vi "Plot Pole-Zero - cascade.vi"(4 "IIR Filter Cluster":T1) -> (1 "Pole-Zero Plot":cluster{dbl[], dbl[]}[](graph))   [LabVIEW 2016]
doc: "Plot the pole-zero diagram of a filter described by its cascade-form IIR filter cluster."
uses:
  <vilib>/Analysis/1siggen.llb/Ramp Pattern by Samples.vi
  <vilib>/Analysis/polynomials.llb/Remove Zero Coefficients (DBL).vi
  <vilib>/Analysis/polynomials.llb/Polynomial Roots (DBL).vi
  <vilib>/Analysis/NI_AALPro.lvlib
  <vilib>/Analysis/NI_AALBase.lvlib
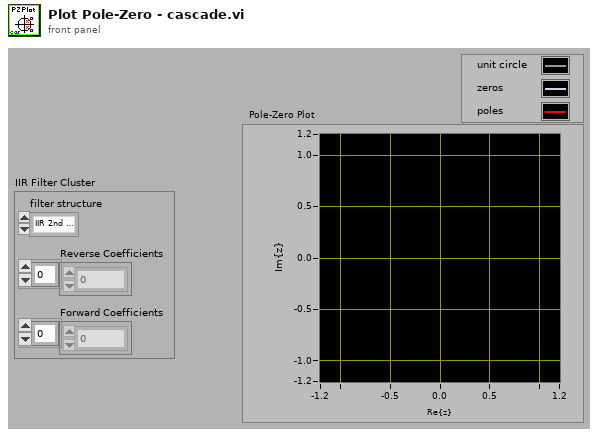
[diagram p1: front panel]
types:
  T1 = cluster{"filter structure":enum32{"IIR 2nd Order", "IIR 4th Order"}, "Reverse Coefficients":dbl[], "Forward Coefficients":dbl[]}
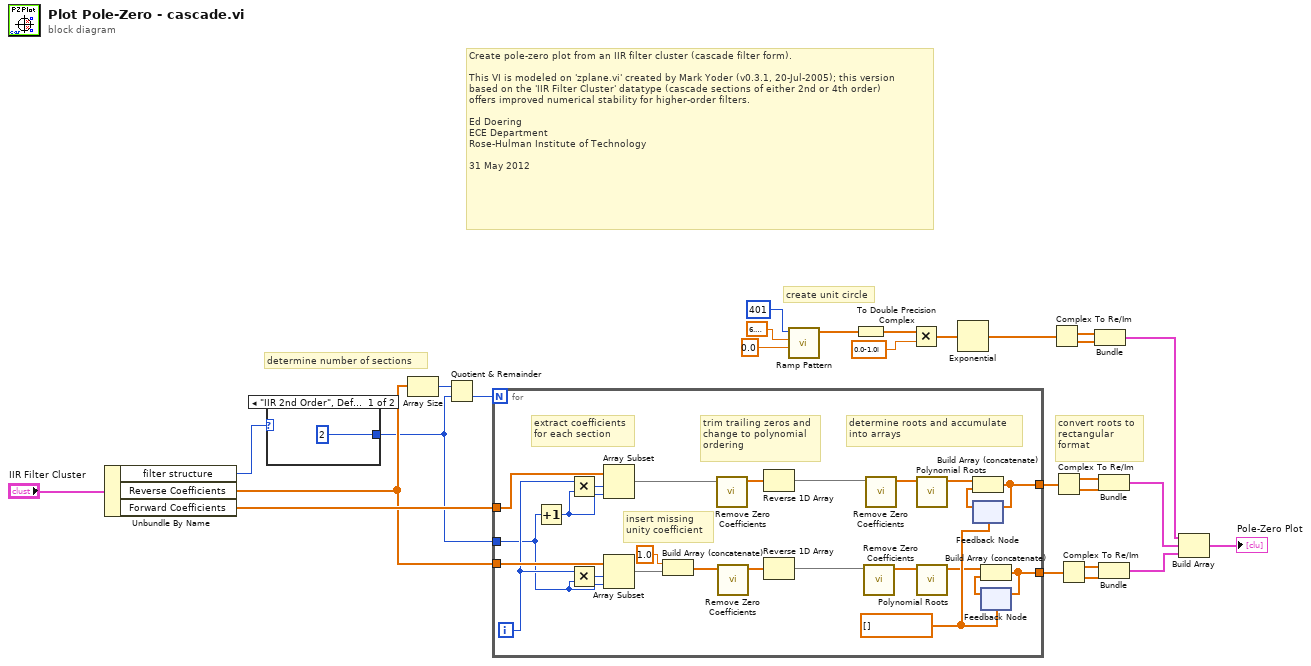
[diagram p0: block diagram]
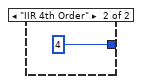
[diagram p2: hidden frame]
diagram:
  # "create unit circle"
  # "Create pole-zero plot from an IIR filter cluster (cascade filter form).\n\nThis VI is modeled on 'zplane.vi' created by Mark Yoder (v0.3.1, 20-Jul-2005); this version\nbased on the 'IIR Filter Cluster' datatype (cascade sections of either 2nd or 4th order)\noffers improved numerical stability for higher-order filters.\n\nEd Doering\nECE Department\nRose-Hulman Institute of Technology\n\n31 May 2012"
  # "convert roots to\nrectangular \nformat"
  # "determine number of sections"
  n1 = Unbundle By Name("IIR Filter Cluster") -> ("filter structure"=w19:enum32{"IIR 2nd Order", "IIR 4th Order"}, "Reverse Coefficients"=w21:dbl[], "Forward Coefficients"=w22:dbl[])
  n2 = case shown="\"IIR 2nd Order\", Default" w19 {
    tunnel: [2 ("y") 4 ("y")] -> w12
    frame "IIR 2nd Order", Default {
    }
    frame "IIR 4th Order" {
    }
  }
  n3 = Array Size(array=w21) -> (size(s)=w23:i32)
  n4 = Quotient & Remainder(x=w23, y=w12) -> (floor(x/y)=w20:i32)  [unwired: 1 out]
  n5 = for {
    N: w20 -> [_]
    tunnel: w22 -> [w52]
    tunnel: w21 -> [w50]
    tunnel: [w44] -> w18
    tunnel: [w43] -> w15
    tunnel: w12 -> [w38]
    i -> [w42]
    w45 = cdb[] []
    # "determine roots and accumulate\ninto arrays"
    # "trim trailing zeros and\nchange to polynomial\nordering"
    # "insert missing\nunity coefficient"
    # "extract coefficients\nfor each section"
    n6 = Increment(x=w38) -> (x+1=w41:i32)
    n7 = Multiply(x=w42, y=w41) -> (x*y=w53:i32)
    n8 = Multiply(x=w42, y=w38) -> (x*y=w51:i32)
    n9 = Array Subset(array=w52, index=w53, length=w41) -> (w33:dbl[])
    n10 = Array Subset(array=w50, index=w51, length=w38) -> (w48:dbl[])
    n11 = Build Array (concatenate)(1.0 ("element"), w48) -> (w30:dbl[])
    n12 = call-poly <vilib>:"Remove Zero Coefficients.vi"("P(x) In"=w33) -> ("P(x) Out"=w32:dbl[])  [unwired: 8 in, 2 out]
    n13 = call-poly <vilib>:"Remove Zero Coefficients.vi"("P(x) In"=w30) -> ("P(x) Out"=w31:dbl[])  [unwired: 8 in, 2 out]
    n14 = Reverse 1D Array(array=w32) -> (reversed array=w35:dbl[])
    n15 = Reverse 1D Array(array=w31) -> (reversed array=w34:dbl[])
    n16 = call-poly <vilib>:"Remove Zero Coefficients.vi"("P(x) In"=w34) -> ("P(x) Out"=w36:dbl[])  [unwired: 8 in, 2 out]
    n17 = call-poly <vilib>:"Remove Zero Coefficients.vi"("P(x) In"=w35) -> ("P(x) Out"=w37:dbl[])  [unwired: 8 in, 2 out]
    n18 = call-poly <vilib>:"Polynomial Roots.vi"("P(x)"=w37) -> ("Roots"=w40:cdb[])  [unwired: 9 in, 1 out]
    n19 = call-poly <vilib>:"Polynomial Roots.vi"("P(x)"=w36) -> ("Roots"=w39:cdb[])  [unwired: 9 in, 1 out]
    n20 = feedback #1(w45) -> (w47:cdb[])
    n21 = Build Array (concatenate)(w40, w47) -> (w44:cdb[])
    n22 = feedback-in #1(w44) -> ()
    n23 = feedback #2(w45) -> (w46:cdb[])
    n24 = Build Array (concatenate)(w39, w46) -> (w43:cdb[])
    n25 = feedback-in #2(w43) -> ()
  }
  n26 = call-poly <vilib>:"Ramp Pattern.vi"("start"=0.0, "end"=6.283185307179586, "samples"=401) -> ("Ramp Pattern"=w6:dbl[])  [unwired: 7 in, 1 out]
  n27 = To Double Precision Complex(1:w6) -> (0:w7:cdb[])
  n28 = Multiply(x=w7, y=cdb 0.0-1.0i) -> (x*y=w9:cdb[])
  n29 = Exponential(1:w9) -> (0:w5:cdb[])
  n30 = Complex To Re/Im(x + iy=w5) -> (x=w3:dbl[], y=w4:dbl[])
  n31 = Complex To Re/Im(x + iy=w18) -> (x=w17:dbl[], y=w16:dbl[])
  n32 = Complex To Re/Im(x + iy=w15) -> (x=w14:dbl[], y=w13:dbl[])
  n33 = Bundle(w3, w4) -> (w2:cluster{dbl[], dbl[]})  [unwired: 1 in]
  n34 = Bundle(w17, w16) -> (w26:cluster{dbl[], dbl[]})  [unwired: 1 in]
  n35 = Bundle(w14, w13) -> (w27:cluster{dbl[], dbl[]})  [unwired: 1 in]
  n36 = Build Array(w2, w26, w27) -> (→"Pole-Zero Plot":cluster{dbl[], dbl[]}[])
